vi "Initialize N Pins.vi"(8 "error in":errorcluster, 9 "Initialize_Info":T1, 10 "pin or relay names":string[](array[string]), 11 "measure call context in":refnum<class "Measure Call Context.lvclass">) -> (0 "error out":errorcluster, 1 "instrument object":refnum<class "Abstract_Instrument.lvclass">[](array[class]), 2 "session reservation out":refnum<class "Session Reservation.lvclass">, 3 "measure call context out":refnum<class "Measure Call Context.lvclass">)   [LabVIEW 2021, in "Abstract_Instrument.lvclass"]
uses:
  Abstract_Instrument.lvclass
  controls/Initialize_Info.ctl
  <vilib>/Plug-In SDKs/Clients/Session Management V1/Session Reservation/Initialize and Close Session Behavior.ctl
  <vilib>/Plug-In SDKs/Measurements/Measure Call Context/Measure Call Context.lvclass
  <vilib>/Plug-In SDKs/Clients/Session Management V1/Session Reservation/Session Reservation.lvclass
  <vilib>/Plug-In SDKs/Measurements/Measure Call Context/Reserve Sessions - NPin.vi
  Reusables/Get Pin Information.lvlib
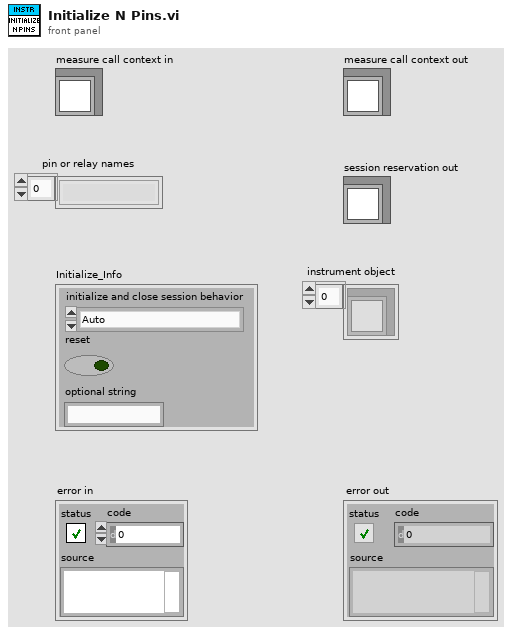
[diagram p1: front panel]
types:
  T1 = typedef "Abstract_Instrument.lvclass/Initialize_Info.ctl" = cluster{"initialize and close session behavior":T2, "reset":bool, "optional string":string}
  T2 = typedef "NI Session Management V1 Client.lvlib/Session Reservation.lvclass/Initialize and Close Session Behavior.ctl" = enum16{"Auto", "Initialize and Close", "Attach and Detach", "Initialize and Detach", "Attach and Close"}
  T3 = typedef "ni.measurementlink.sessionmanagement.v1.api.lvlib/ni_measurementlink_sessionmanagement_v1_ChannelMapping.ctl" = cluster{"pin_or_relay_name":string, "site":i32, "channel":string, "multiplexer_resource_name":string, "multiplexer_route":string}
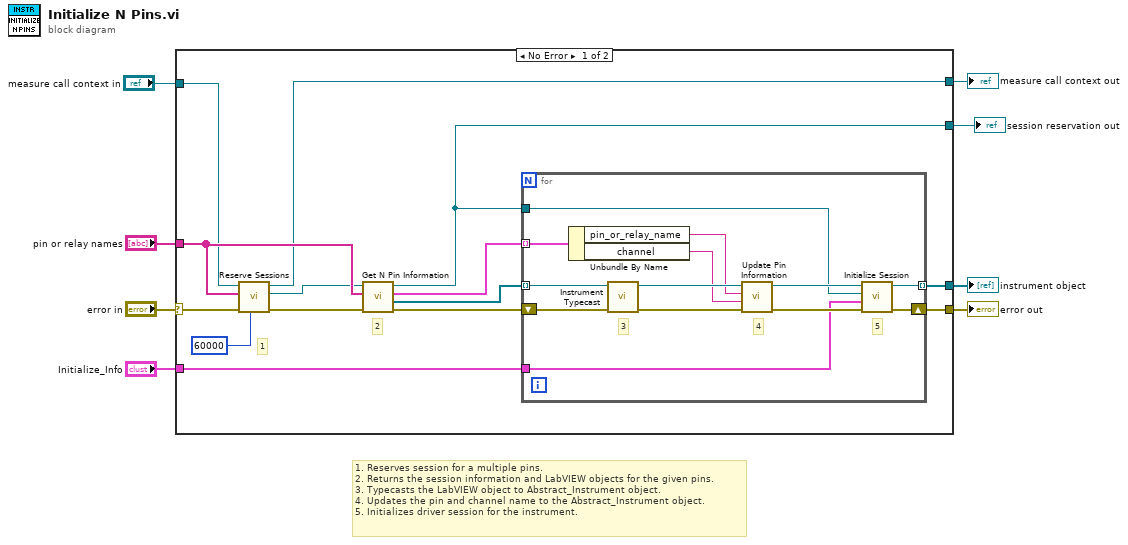
[diagram p0: block diagram]
diagram:
  # "1. Reserves session for a multiple pins.\n2. Returns the session information and LabVIEW objects for the given pins.\n3. Typecasts the LabVIEW object to Abstract_Instrument object.\n4. Updates the pin and channel name to the Abstract_Instrument object.\n5. Initializes driver session for the instrument."
  n1 = case shown="No Error" "error in" {
    selector: "error in" -> [w18 w37]
    tunnel: [w19 w37] -> w8
    tunnel: "pin or relay names" -> [w15 _]
    tunnel: [w14 _] -> w5
    tunnel: "Initialize_Info" -> [w13 _]
    tunnel: "measure call context in" -> [w12 w36]
    tunnel: [w11 w36] -> w2
    tunnel: [w9 _] -> w1
    frame No Error {
      # "2"
      # "1"
      n2 = call-poly <vilib>:"Reserve Sessions.vi"("timeout (ms)"=60000, "error in"=w18, "pin or relay names"=w15, "measurement context in"=w12) -> ("error out"=w17:errorcluster, "session reservation out"=w10:refnum<class "Session Reservation.lvclass">, "measurement context out"=w11:refnum<class "Measure Call Context.lvclass">)  [unwired: 5 in]
      n3 = call "Get N Pin Information.vi"("error in"=w17, "pin or relay names"=w15, "session reservation"=w10) -> ("error out"=w22:errorcluster, "pin instruments"=w21:refnum<class>[], "channel_mappings"=w20:T3[], "session reservation out"=w9:refnum<class "Session Reservation.lvclass">)  [unwired: 5 in]
      n4 = for {
        shift-right: [w26] -> w19
        shift-left: w22 -> [w35]
        tunnel: w21 -> [w24] mode=indexing
        tunnel: w20 -> [w34] mode=indexing
        tunnel: w9 -> [w27]
        tunnel: w13 -> [w23]
        tunnel: [w25] -> w14 mode=indexing
        # "5"
        # "4"
        # "3"
        n5 = Unbundle By Name(w34) -> ("pin_or_relay_name"=w31:string, "channel"=w30:string)
        n6 = call "Instrument Typecast.vi"("error in (no error)"=w35, "pin instrument"=w24) -> ("error out"=w33:errorcluster, "instrument object"=w32:refnum<class "Abstract_Instrument.lvclass">)  [unwired: 8 in]
        n7 = call "Update Pin Information.vi"("error in"=w33, "channel"=w30, "pin_name"=w31, "instrument object in"=w32) -> ("error out"=w29:errorcluster, "instrument object out"=w28:refnum<class "Abstract_Instrument.lvclass">)  [unwired: 6 in]
        n8 = call-dynamic "Initialize Session.vi"("error in (no error)"=w29, "Initialize_Info"=w23, "session reservation in"=w27, "Abstract_Instrument in"=w28) -> ("error out"=w26:errorcluster, "Abstract_Instrument out"=w25:refnum<class "Abstract_Instrument.lvclass">)  [unwired: 6 in]
      }
    }
    frame Error {
    }
  }
  "error out" <- w8
  "instrument object" <- w5
  "measure call context out" <- w2
  "session reservation out" <- w1
